vi "ServiceLocationPool_DiscoveryServiceUnavailable_GetUncachedLocation_ReturnsError.vi"(8 "error in (no error)":errorcluster) -> (0 "error out":errorcluster, 2 "result":string, 3 "pass":bool)   [LabVIEW 2020, in "MeasurementServerTests.lvlib"]
uses:
  MeasurementServerTests.lvlib
  Runtime/MeasurementLink Discovery Client/RPC Messages/ni_measurementlink_discovery_v1_ResolveServiceRequest.ctl
  Runtime/MeasurementLink gRPC Utilities/TypeDefs/Service Location FGV Action.ctl
  Runtime/MeasurementLink gRPC Utilities/MeasurementLink gRPC Utilities.lvlib
  Runtime/MeasurementLink Discovery Client/MeasurementLink Discovery Client.lvlib
  Runtime/MeasurementLink Measurement Server/MeasurementLink Measurement Server.lvlib
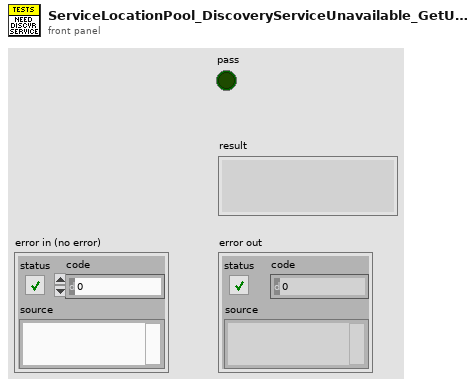
[diagram p1: front panel]
types:
  T1 = typedef "MeasurementLink gRPC Utilities.lvlib/Service Location FGV Action.ctl" = enum16{"Get Service Location", "Clear Cache"}
  T2 = typedef "MeasurementLink Discovery Client.lvlib/ni_measurementlink_discovery_v1_ResolveServiceRequest.ctl" = cluster{"provided_interface":string, "service_class":string}
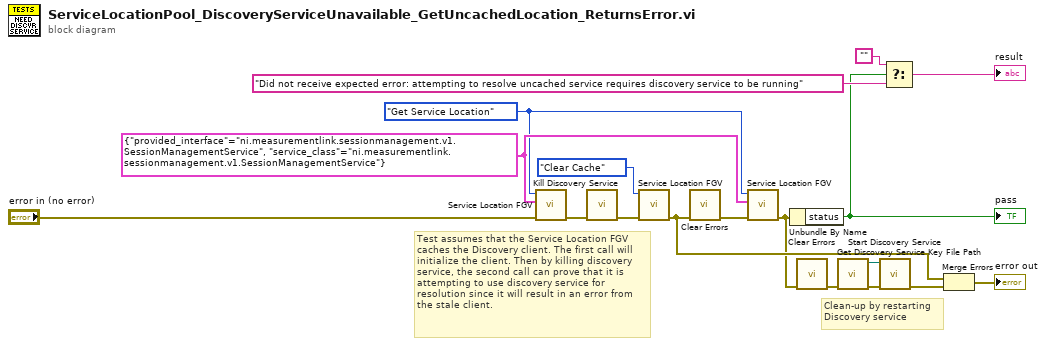
[diagram p0: block diagram]
diagram:
  w1 = Service_Location_FGV_Action."Get Service Location" ("Action")
  w14 = T2 {"provided_interface"="ni.measurementlink.sessionmanagement.v1.SessionManagementService", "service_class"="ni.measurementlink.sessionmanagement.v1.SessionManagementService"} ("Resolve Service Request")
  # "Clean-up by restarting\nDiscovery service"
  # "Test assumes that the Service Location FGV\ncaches the Discovery client. The first call will\ninitialize the client. Then by killing discovery\nservice, the second call can prove that it is\nattempting to use discovery service for\nresolution since it will result in an error from\nthe stale client."
  n1 = call "Service Location FGV.vi"("error in"="error in (no error)", "Resolve Service Request"=w14, "Action"=w1) -> ("error out"=w16:errorcluster)  [unwired: 7 in, 1 out]
  n2 = call "Kill Discovery Service.vi"("error in"=w16) -> ("error out"=w13:errorcluster)  [unwired: 10 in]
  n3 = call "Service Location FGV.vi"("error in"=w13, "Action"=Service_Location_FGV_Action."Clear Cache") -> ("error out"=w5:errorcluster)  [unwired: 8 in, 1 out]
  n4 = call <vilib>:"Clear Errors.vi"("error in (no error)"=w5) -> ("error out"=w4:errorcluster)  [unwired: 5 in, 1 out]
  n5 = call "Service Location FGV.vi"("error in"=w4, "Resolve Service Request"=w14, "Action"=w1) -> ("error out"=w3:errorcluster)  [unwired: 7 in, 1 out]
  n6 = Unbundle By Name(w3) -> ("status"=w10:bool)
  "pass" <- w10
  n7 = call <vilib>:"Clear Errors.vi"("error in (no error)"=w3) -> ("error out"=w2:errorcluster)  [unwired: 5 in, 1 out]
  n8 = call "Get Discovery Service Key File Path.vi"("error in (no error)"=w2) -> ("error out"=w9:errorcluster, "key file path"=w8:path)  [unwired: 9 in]
  n9 = call "Start Discovery Service.vi"("error in"=w9, "key file path"=w8) -> ("error out"=w7:errorcluster)  [unwired: 9 in]
  n10 = Select(t="", s=w10, f="Did not receive expected error: attempting to resolve uncached service requires discovery service to be running") -> (s? t:f=→"result":string)
  n11 = Merge Errors(w5, w7) -> (→"error out":errorcluster)
